vi "StartUpSequence.vi"(2 "error in":errorcluster, 3 "Cluster 2":T2) -> (0 "error out":errorcluster)   [LabVIEW 2011]
uses:
  Utilities/controls/ctlSeqFNs_AVTGuppy.ctl
  Utilities/controls/ctlSeqFNs_Scanner.ctl
  Utilities/controls/ctlSeqFNs_CTIOTF.ctl
  Utilities/controls/ctlSeqFNs_Andor.ctl
  Utilities/controls/ctlSeqFNs_Koheras.ctl
  Utilities/controls/ctlSeqFNs_Heidenhain.ctl
  <vilib>/userDefined/High Color/IMAQdx.ctl
  Utilities/controls/ctlSeqFNs_Main.ctl
  Utilities/controls/ctlSeqFNs_PCDeviceInit.ctl
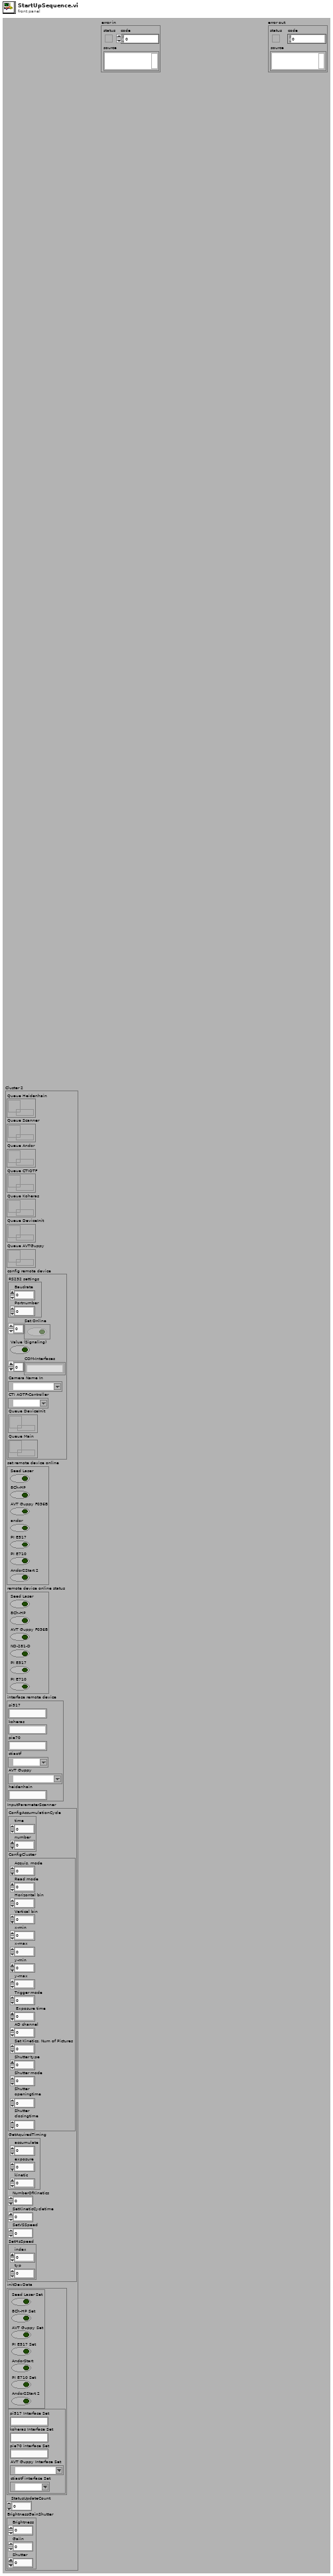
[diagram p1: front panel]
types:
  T1 = typedef "IMAQdx.ctl" = refnum<k21>
  T2 = cluster{"Queue Heidenhain":refnum<queue>, "Queue Scanner":refnum<queue>, "Queue Andor":refnum<queue>, "Queue CTIOTF":refnum<queue>, "Queue Koheras":refnum<queue>, "Queue DeviceInit":refnum<queue>, "Queue AVTGuppy":refnum<queue>, "config remote device":cluster{"RS232 settings":cluster{"Baudrate":u16, "Portnumber":i32}, "Set Online":bool[], "Value (Signaling)":bool, "COM-Interfaces":string[], "Camera Name In":T1, "CTI AOTF-Controller":refnum<visa-resource-name>, "Queue DeviceInit":refnum<queue>, "Queue Main":refnum<queue>}, "set remote device online":cluster{"Seed Laser":bool, "8Ch-HP":bool, "AVT Guppy F036B":bool, "andor":bool, "PI E517":bool, "PI E710":bool, "Andor2Start 2":bool}, "remote device online status":cluster{"Seed Laser":bool, "8Ch-HP":bool, "AVT Guppy F036B":bool, "ND-281-D":bool, "PI E517":bool, "PI E710":bool}, "interface remote device":cluster{"pi517":string, "koheras":string, "pie70":string, "ctiaotf":refnum<visa-resource-name>, "AVT Guppy":T1, "heidenhain":string}, "InputParameterScanner":cluster{"ConfigAccumulationCycle":cluster{"time":sgl, "number":i32}, "ConfigCluster":cluster{"Acquis. mode":u16, "Read mode":u16, "Horizontal bin":i32, "Vertical bin":i32, "x-min":i32, "x-max":i32, "y-min":i32, "y-max":i32, "Trigger mode":u16, " Exposure time":sgl, "AD channel":i32, "Set Kinetics, Num of Pictures":i32, "Shutter type":u16, "Shutter mode":u16, "Shutter\nopeningtime":i32, "Shutter\nclosingtime":i32}, "GetAquiredTiming":cluster{"accumulate":sgl, "exposure":sgl, "kinetic":sgl}, "NumberOfKinetics":i32, "SetKineticCycletime":sgl, "SetVSSpeed":i32, "SetHsSpeed":cluster{"index":i32, "typ":i32}}, "initDevData":cluster{cluster{"Seed Laser Set":bool, "8Ch-HP Set":bool, "AVT Guppy Set":bool, "PI E517 Set":bool, "AndorStart":bool, "PI E710 Set":bool, "Andor2Start 2":bool}, cluster{"pi517 Interface Set":string, "koheras Interface Set":string, "pie70 interface Set":string, "AVT Guppy Interface Set":T1, "ctiaotf interface Set":refnum<visa-resource-name>}}, "StatusUpdateCount":dbl, "BrightnessGainShutter":cluster{"Brightness":i32, "Gaiin":i32, "Shutter":i32}}
  T3 = typedef "ctlSeqFNs_Heidenhain.ctl" = enum16{"ERROR", "INIT", "Initialization", "Configuration", "Measurement", "Shutdown", "IDLE", "EXIT"}
  T4 = typedef "ctlSeqFNs_Koheras.ctl" = enum16{"ERROR", "INIT", "Initialization", "Configuration", "Measurement", "Shutdown", "IDLE", "EXIT"}
  T5 = typedef "ctlSeqFNs_Andor.ctl" = enum16{"ERROR", "INIT", "Initialization", "Configuration", "Measurement", "Shutdown", "IDLE", "EXIT"}
  T6 = typedef "ctlSeqFNs_CTIOTF.ctl" = enum16{"ERROR", "INIT", "Initialization", "Configuration", "Measurement", "Shutdown", "IDLE", "EXIT"}
  T7 = typedef "ctlSeqFNs_Scanner.ctl" = enum16{"ERROR", "INIT", "Initialization", "Configuration", "Measurement", "Shutdown", "IDLE", "EXIT"}
  T8 = typedef "ctlSeqFNs_AVTGuppy.ctl" = enum16{"ERROR", "INIT", "Initialization", "Configuration", "Measurement", "Shutdown", "IDLE", "EXIT"}
  T9 = cluster{"pi517 Interface Set":string, "pie70 interface Set":string, "PI E710":bool, "PI E517":bool}
  T10 = cluster{"Koheras":bool, "AOTF":bool, "ctiaotf interface Set":refnum<visa-resource-name>, "koheras Interface Set":string}
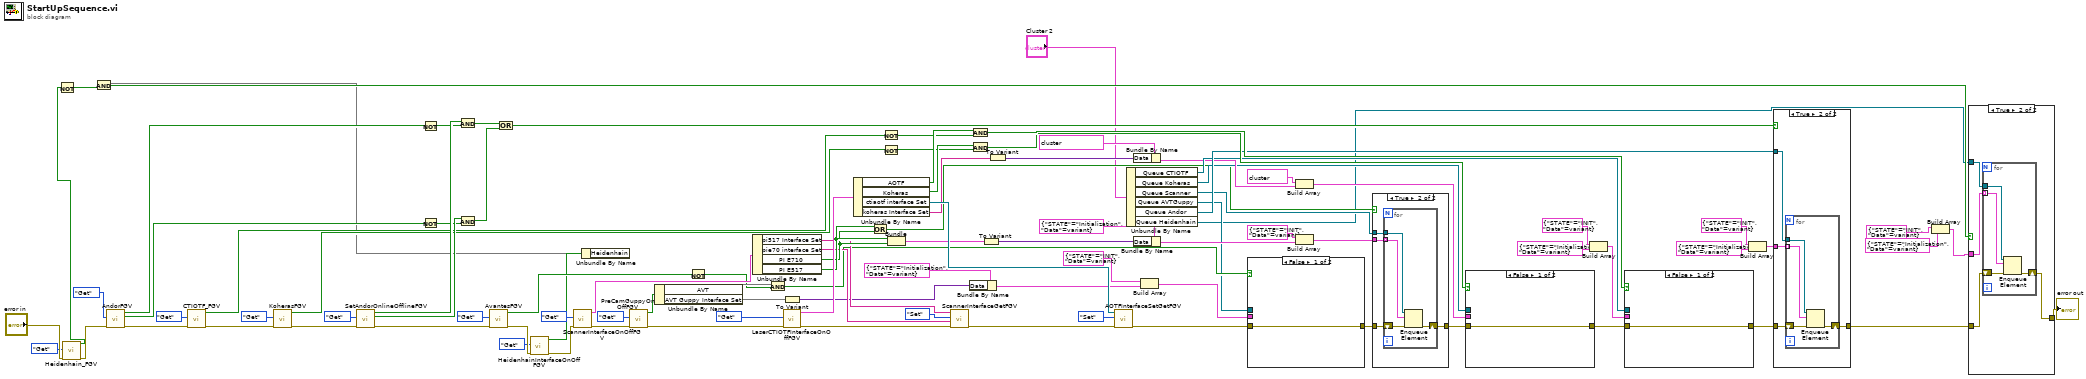
[diagram p0: block diagram]
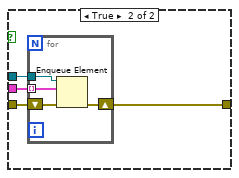
[diagram p4: hidden frame]
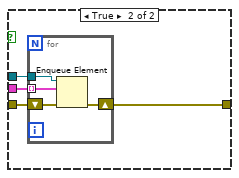
[diagram p5: hidden frame]
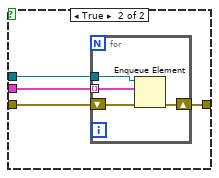
[diagram p7: hidden frame]
diagram:
  n1 = call "Heidenhain_FGV.vi"("error in"="error in", "Set_Get"=enum16{"Set", "Get"}."Get") -> ("error out"=w17:errorcluster, "Get"=w1:bool)  [unwired: 8 in]
  n2 = Not(x=w1) -> (.not. x?=w15:bool)
  n3 = call "AndorFGV.vi"("error in"=w17, "Set_Get"=enum16{"Set", "Get"}."Get") -> ("error out"=w78:errorcluster, "andor 1"=w69:bool, "andor 0"=w59:bool)  [unwired: 7 in]
  n4 = call "CTIOTF_FGV.vi"("error in"=w78, "Set_Get"=enum16{"Set", "Get"}."Get") -> ("error out"=w79:errorcluster, "aotfGet"=w57:bool)  [unwired: 8 in]
  n5 = call "KoherasFGV.vi"("error in"=w79, "Set_Get"=enum16{"Set", "Get"}."Get") -> ("error out"=w96:errorcluster, "Get"=w55:bool)  [unwired: 8 in]
  n6 = call "SetAndorOnlineOfflineFGV.vi"("error in"=w96, "Set_Get"=enum16{"Set", "Get"}."Get") -> ("error out"=w97:errorcluster, "andor 1"=w100:bool, "andor 0"=w99:bool)  [unwired: 7 in]
  n7 = Not(x=w59) -> (.not. x?=w60:bool)
  n8 = Not(x=w69) -> (.not. x?=w68:bool)
  n9 = And(x=w99, y=w60) -> (x .and. y?=w71:bool)
  n10 = And(x=w100, y=w68) -> (x .and. y?=w72:bool)
  n11 = call "AvantesFGV.vi"("error in"=w97, "Set_Get"=enum16{"Set", "Get"}."Get") -> ("error out"=w13:errorcluster, "Get"=w61:bool)  [unwired: 8 in]
  n12 = Or(x=w71, y=w72) -> (x .or. y?=w70:bool)
  n13 = call "HeidenhainInterfaceOnOffFGV.vi"("error in"=w13, "Set_Get"=enum16{"Set", "Get"}."Get") -> ("error out"=w14:errorcluster, "out"=w11:bool)  [unwired: 8 in]
  n14 = call "ScannerInterfaceOnOffFGV.vi"("error in"=w14, "Set_Get"=enum16{"Set", "Get"}."Get") -> ("error out"=w75:errorcluster, "ScannerInterfaceOUT"=w83:T9)  [unwired: 8 in]
  n15 = Unbundle By Name(w11) -> ("Heidenhain"=w2)
  n16 = And(x=w2, y=w15) -> (x .and. y?=w10:bool)
  n17 = call "PreCamGuppyOnOffFGV.vi"("error in"=w75, "Set_Get"=enum16{"Set", "Get"}."Get") -> ("error out"=w76:errorcluster, "out"=w88:bool)  [unwired: 8 in]
  n18 = Unbundle By Name(w88) -> ("AVT"=w90, "AVT Guppy Interface Set"=w89)
  n19 = Not(x=w61) -> (.not. x?=w62:bool)
  n20 = Unbundle By Name(w83) -> ("pi517 Interface Set"=w84:string, "pie70 interface Set"=w85:string, "PI E710"=w86:bool, "PI E517"=w87:bool)
  n21 = And(x=w90, y=w62) -> (x .and. y?=w49:bool)
  n22 = call "LaserCTIOTFInterfaceOnOffFGV.vi"("error in"=w76, "Set_Get"=enum16{"Set", "Get"}."Get") -> ("error out"=w77:errorcluster, "LaserCtiotfInterfaceOnOffOUT"=w91:T10)  [unwired: 8 in]
  n23 = To Variant(anything=w89) -> (Variant=w20:variant)
  n24 = Unbundle By Name(w91) -> ("AOTF"=w95:bool, "Koheras"=w94:bool, "ctiaotf interface Set"=w93:refnum<visa-resource-name>, "koheras Interface Set"=w92:string)
  n25 = Or(x=w87, y=w86) -> (x .or. y?=w28:bool)
  n26 = Not(x=w57) -> (.not. x?=w58:bool)
  n27 = Not(x=w55) -> (.not. x?=w56:bool)
  n28 = Bundle("PI E517"=w87, "PI E710"=w86) -> (w54:cluster{"PI E517":bool, "PI E710":bool})  [unwired: 1 in]
  n29 = call "ScannerInterfaceGetFGV.vi"("error in"=w77, "pie70 interface Set"=w85, "FGV_Control"=enum16{"Set", "Get"}."Set", "pi517 Interface Set"=w84) -> ("error out"=w66:errorcluster)  [unwired: 5 in, 2 out]
  n30 = Bundle By Name(cluster=cluster{"STATE":T8, "Data":variant} {"STATE"=enum."Initialization", "Data"=variant} ("element"), "Data"=w20) -> (w22:cluster{"STATE":T8, "Data":variant})
  n31 = And(x=w95, y=w58) -> (x .and. y?=w47:bool)
  n32 = And(x=w94, y=w56) -> (x .and. y?=w45:bool)
  n33 = To Variant(anything=w54) -> (Variant=w53:variant)
  n34 = To Variant(anything=w92) -> (Variant=w21:variant)
  n35 = call "AOTFInterfaceSetGetFGV.vi"("error in"=w66, "FGV_Control"=enum16{"Set", "Get"}."Set", "ctiaotf interface Set"=w93) -> ("error out"=w67:errorcluster)  [unwired: 7 in, 1 out]
  n36 = Unbundle By Name("Cluster 2") -> ("Queue CTIOTF"=w35:refnum<queue>, "Queue Koheras"=w32:refnum<queue>, "Queue Scanner"=w27:refnum<queue>, "Queue AVTGuppy"=w25:refnum<queue>, "Queue Andor"=w39:refnum<queue>, "Queue Heidenhain"=w6:refnum<queue>)
  n37 = Bundle By Name(cluster=cluster{"Data":variant, "FGV_Control":T4} {"Data"=variant, "FGV_Control"=enum."Initialization"} ("element"), "Data"=w21) -> (w33:cluster{"Data":variant, "FGV_Control":T4})
  n38 = Bundle By Name(cluster=cluster{"STATE":T7, "Data":variant} {"STATE"=enum."Initialization", "Data"=variant} ("element"), "Data"=w53) -> (w52:cluster{"STATE":T7, "Data":variant})
  n39 = Build Array(cluster{"STATE":T8, "Data":variant} {"STATE"=enum."INIT", "Data"=variant} ("element"), w22) -> (w24:cluster{"STATE":T8, "Data":variant}[])
  n40 = case shown="False" w49 {
    tunnel: [w101 w105] -> w26
    tunnel: w67 -> [w101 w104]
    tunnel: w24 -> [_ w103]
    tunnel: w25 -> [_ w102]
    frame False {
    }
    frame True {
      n41 = for {
        tunnel: w102 -> [w109]
        shift-right: [w107] -> w105
        shift-left: w104 -> [w108]
        tunnel: w103 -> [w106] mode=indexing
        n42 = Enqueue Element(queue=w109, element=w106, error in (no error)=w108) -> (error out=w107:errorcluster)  [unwired: 1 in, 2 out]
      }
    }
  }
  n43 = Build Array(cluster{"Data":variant, "FGV_Control":T4} {"Data"=variant, "FGV_Control"=enum."INIT"} ("element"), w33) -> (w34:cluster{"Data":variant, "FGV_Control":T4}[])
  n44 = Build Array(cluster{"STATE":T7, "Data":variant} {"STATE"=enum."INIT", "Data"=variant} ("element"), w52) -> (w29:cluster{"STATE":T7, "Data":variant}[])
  n45 = case shown="True" w28 {
    tunnel: [w110 w114] -> w31
    tunnel: w26 -> [w110 w113]
    tunnel: w29 -> [_ w112]
    tunnel: w27 -> [_ w111]
    frame False {
    }
    frame True {
      n46 = for {
        tunnel: w111 -> [w118]
        shift-right: [w116] -> w114
        shift-left: w113 -> [w117]
        tunnel: w112 -> [w115] mode=indexing
        n47 = Enqueue Element(queue=w118, element=w115, error in (no error)=w117) -> (error out=w116:errorcluster)  [unwired: 1 in, 2 out]
      }
    }
  }
  n48 = case shown="False" w45 {
    tunnel: [w119 w123] -> w38
    tunnel: w31 -> [w119 w122]
    tunnel: w34 -> [_ w121]
    tunnel: w32 -> [_ w120]
    frame False {
    }
    frame True {
      n49 = for {
        tunnel: w120 -> [w127]
        shift-right: [w125] -> w123
        shift-left: w122 -> [w126]
        tunnel: w121 -> [w124] mode=indexing
        n50 = Enqueue Element(queue=w127, element=w124, error in (no error)=w126) -> (error out=w125:errorcluster)  [unwired: 1 in, 2 out]
      }
    }
  }
  n51 = Build Array(cluster{"STATE":T6, "Data":variant} {"STATE"=enum."INIT", "Data"=variant} ("element"), cluster{"STATE":T6, "Data":variant} {"STATE"=enum."Initialization", "Data"=variant} ("element")) -> (w37:cluster{"STATE":T6, "Data":variant}[])
  n52 = case shown="False" w47 {
    tunnel: [w128 w132] -> w40
    tunnel: w38 -> [w128 w131]
    tunnel: w37 -> [_ w130]
    tunnel: w35 -> [_ w129]
    frame False {
    }
    frame True {
      n53 = for {
        tunnel: w129 -> [w136]
        shift-right: [w134] -> w132
        shift-left: w131 -> [w135]
        tunnel: w130 -> [w133] mode=indexing
        n54 = Enqueue Element(queue=w136, element=w133, error in (no error)=w135) -> (error out=w134:errorcluster)  [unwired: 1 in, 2 out]
      }
    }
  }
  n55 = Build Array(cluster{"STATE":T5, "Data":variant} {"STATE"=enum."INIT", "Data"=variant} ("element"), cluster{"STATE":T5, "Data":variant} {"STATE"=enum."Initialization", "Data"=variant} ("element")) -> (w43:cluster{"STATE":T5, "Data":variant}[])
  n56 = case shown="True" w70 {
    tunnel: [w137 w141] -> w8
    tunnel: w40 -> [w137 w140]
    tunnel: w43 -> [_ w139]
    tunnel: w39 -> [_ w138]
    frame False {
    }
    frame True {
      n57 = for {
        tunnel: w138 -> [w145]
        shift-right: [w143] -> w141
        shift-left: w140 -> [w144]
        tunnel: w139 -> [w142] mode=indexing
        n58 = Enqueue Element(queue=w145, element=w142, error in (no error)=w144) -> (error out=w143:errorcluster)  [unwired: 1 in, 2 out]
      }
    }
  }
  n59 = Build Array(cluster{"STATE":T3, "Data":variant} {"STATE"=enum."INIT", "Data"=variant} ("element"), cluster{"STATE":T3, "Data":variant} {"STATE"=enum."Initialization", "Data"=variant} ("element")) -> (w3:cluster{"STATE":T3, "Data":variant}[])
  n60 = case shown="True" w10 {
    tunnel: [w146 w150] -> w9
    tunnel: w8 -> [w146 w149]
    tunnel: w6 -> [_ w147]
    tunnel: w3 -> [_ w148]
    frame False {
    }
    frame True {
      n61 = for {
        tunnel: w147 -> [w154]
        shift-right: [w152] -> w150
        shift-left: w149 -> [w153]
        tunnel: w148 -> [w151] mode=indexing
        n62 = Enqueue Element(queue=w154, element=w151, error in (no error)=w153) -> (error out=w152:errorcluster)  [unwired: 1 in, 2 out]
      }
    }
  }
  "error out" <- w9
